vi "Teste de resolução.vi"() -> ()   [LabVIEW 2020]
uses:
  <vilib>/vision/NI_Vision_Development_Module.lvlib
panel:
  in  "Pasta das imagens":path
  in  "Fonte das imagens":enum16{"Imagens na pasta", "Câmera"}(ring)
  in  "Resolução":T1(ring)
  in  "Código para rastrear":enum16{"QR Code", "Data Matrix"}(ring)
  in  "Altura":u16(slide)=3036 scale=10.0..3036.0
  in  "Largura":u16(slide)=4024 scale=10.0..4024.0
  in  "Stop (F)":bool
  out "Image Out":T2(plugin-control)
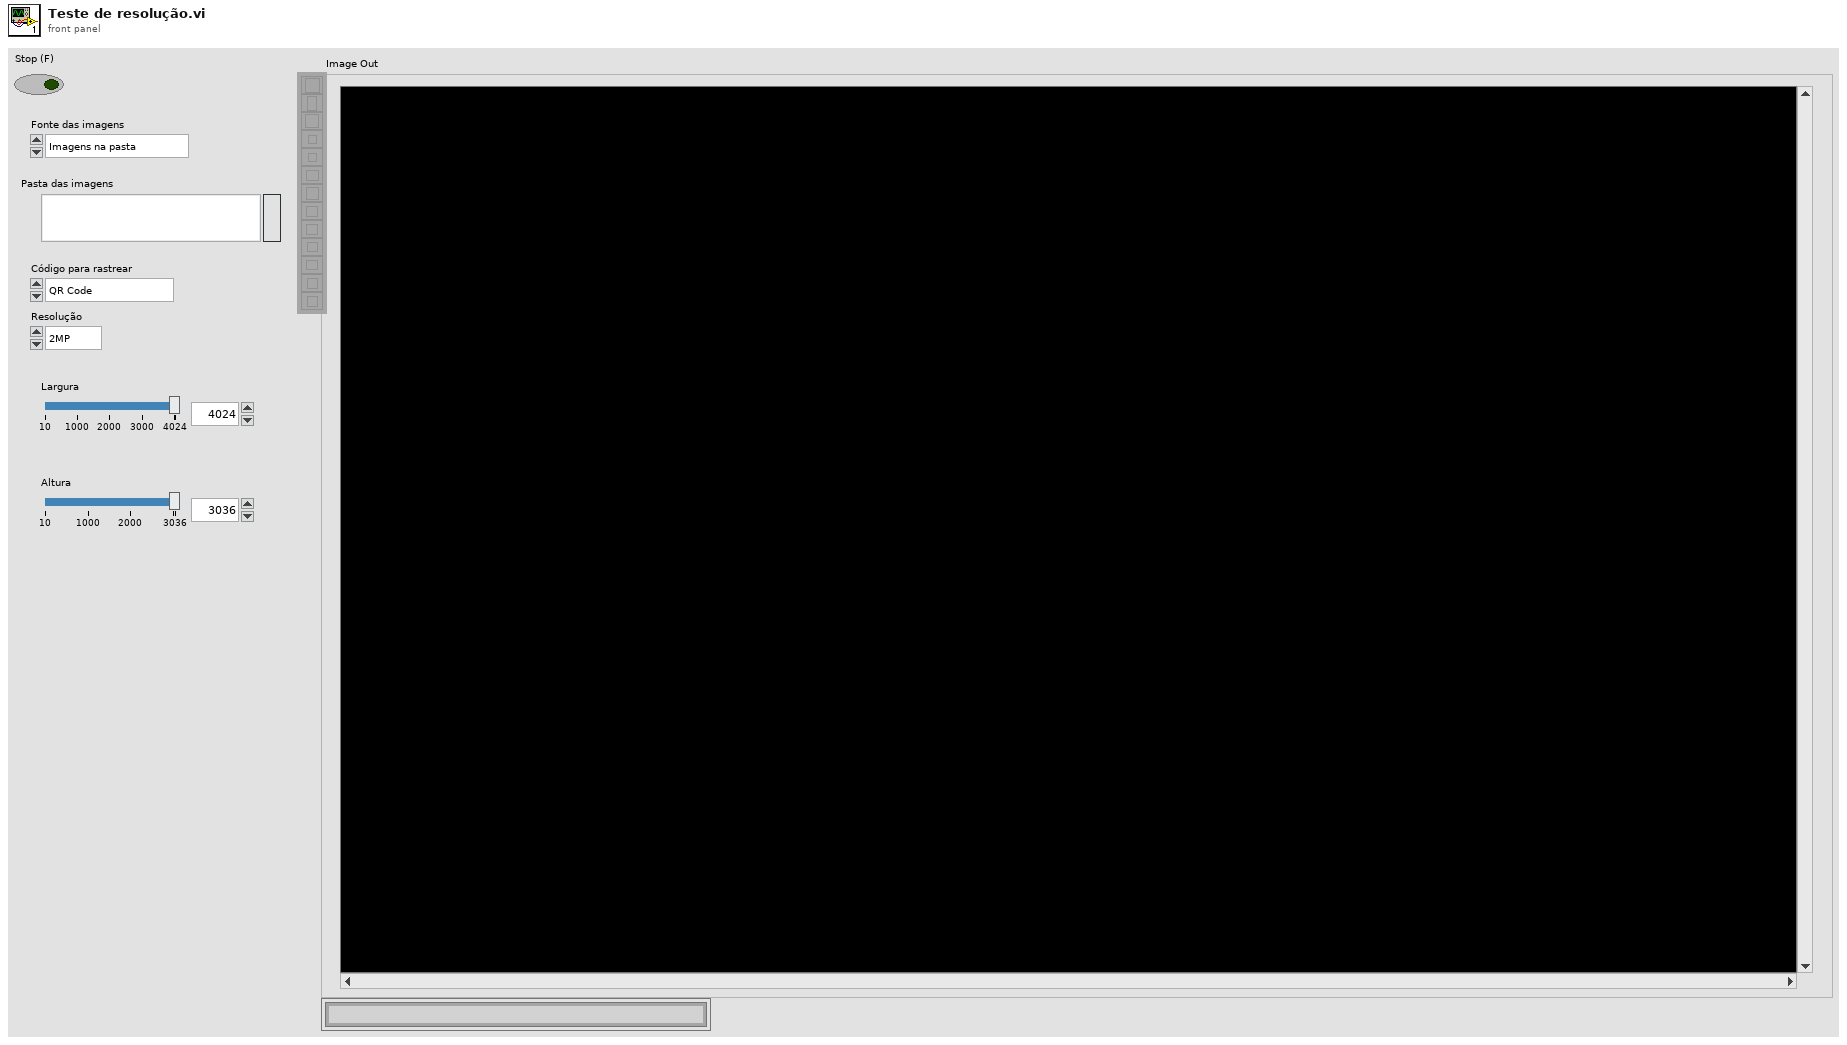
[diagram p1: front panel]
types:
  T1 = enum16{"2MP", "3MP", "5MP", "7MP", "8MP", "10MP", "12MP"}
  T2 = typedef "IMAQ Image.ctl" = refnum<image>
  T3 = cluster{"Global Rectangle":i32[], "Contours":cluster{"Contour Type":u32, "ROI Type":u32, "Points":i32[]}[]}
  T4 = typedef "QR Code Report.ctl" = cluster{"Found?":bool, "Data":string, "Bounding Box":cluster{"x":sgl, "y":sgl}[], "Errors Corrected":u32, "Dimensions (Rows/Cols)":u32, "Version":u32, "QR Model":T5, "Stream Mode":T6, "Barcode Polarity":T7, "Mirrored?":bool, "Append Stream Position":u32, "Size of Append Stream":u32, "First EAN-128 ID":i32, "First Alternate Language ID":i32, "Append Stream ID":u32, "Minimum Edge Strength":u32, "Demodulation Mode":T8, "Cell Sample Size":T9, "Cell Filter Mode":T10}
  T5 = typedef "QR Code Model Type.ctl" = i32
  T6 = typedef "QR Code Stream Mode Type.ctl" = i32
  T7 = typedef "Data Matrix Polarity.ctl" = i32
  T8 = typedef "Demodulation Mode.ctl" = i32
  T9 = typedef "Cell Sample Size.ctl" = i32
  T10 = typedef "Cell Filter Mode.ctl" = i32
  T11 = typedef "Data Matrix Report.ctl" = cluster{"Found?":bool, "Binary?":bool, "Data":string, "Bounding Box":cluster{"x":sgl, "y":sgl}[], "Errors Corrected":u32, "Erasures Corrected":u32, "Aspect Ratio":sgl, "Rows":u32, "Columns":u32, "ECC":T12, "Barcode Polarity":T7, "Cell Fill Percentage":T13, "Border Integrity":sgl, "Mirrored?":bool, "Minimum Edge Strength":u32, "Demodulation Mode":T8, "Cell Sample Size":T9, "Cell Filter Mode":T10, "Iterations":u32}
  T12 = typedef "ECC Type.ctl" = i32
  T13 = typedef "Cell Fill Percentage.ctl" = i32
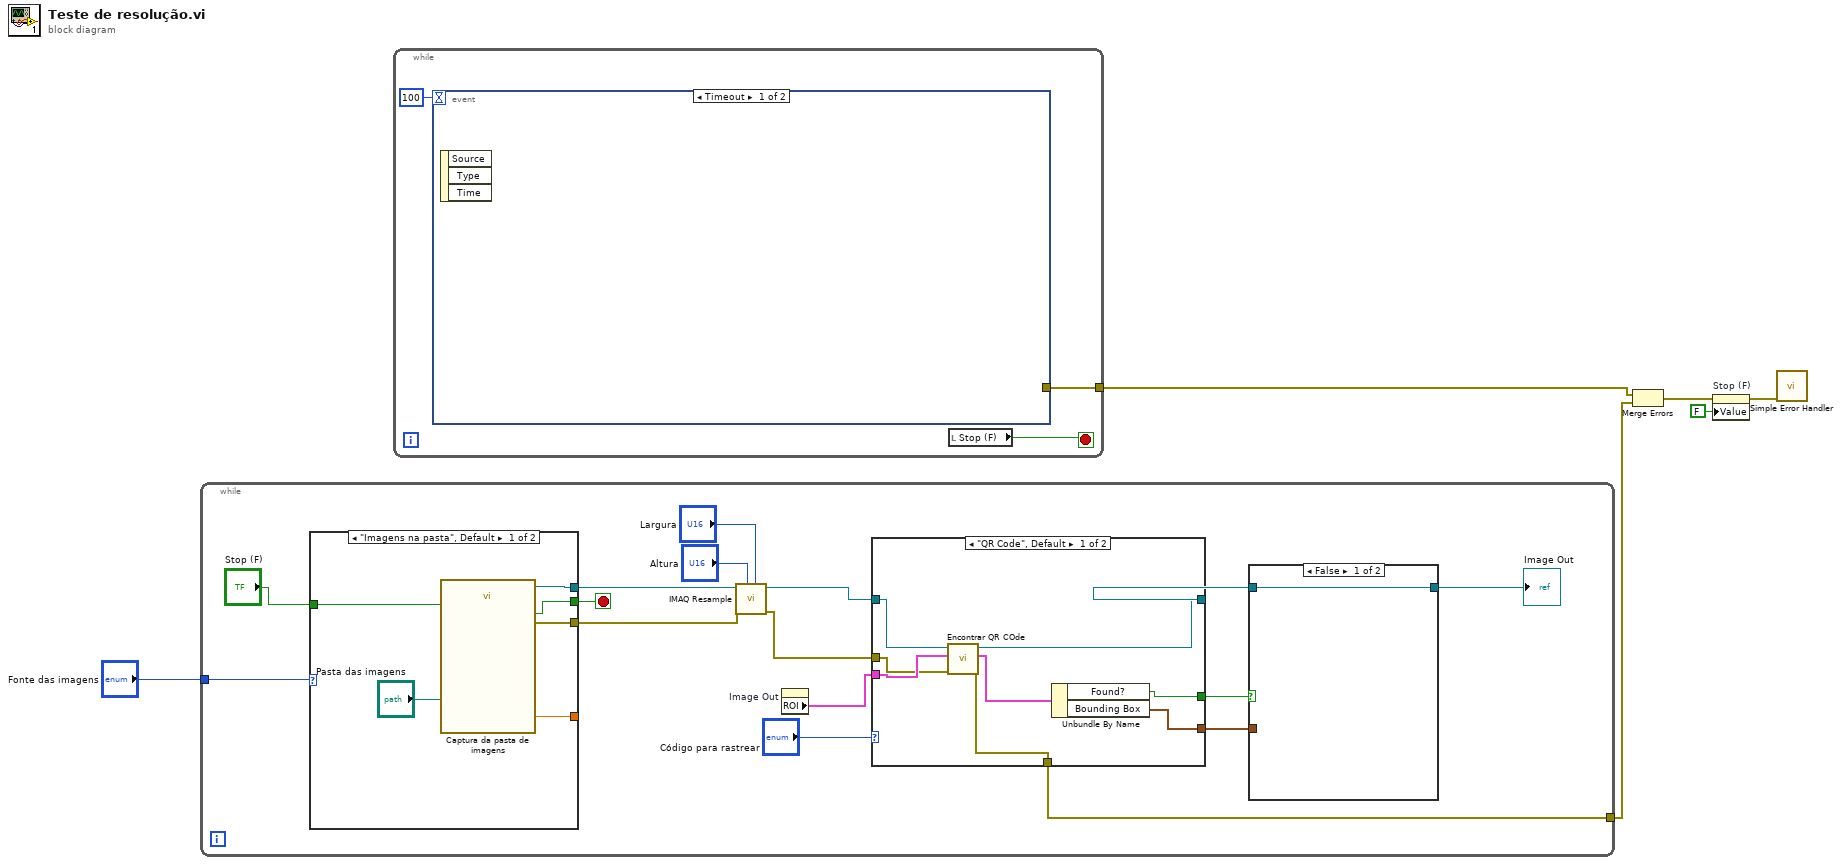
[diagram p0: block diagram]
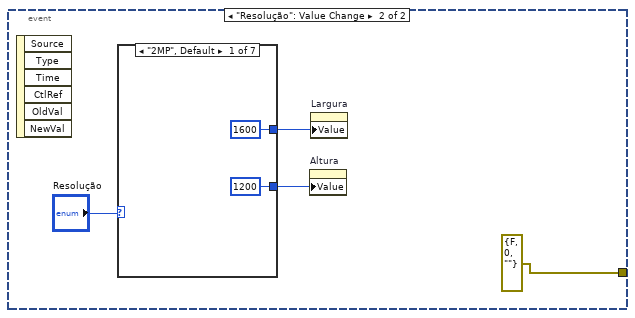
[diagram p2: hidden frame]
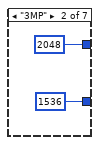
[diagram p3: hidden frame]
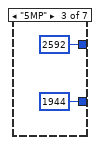
[diagram p4: hidden frame]
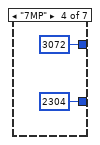
[diagram p5: hidden frame]
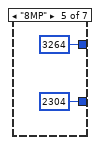
[diagram p6: hidden frame]
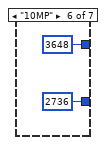
[diagram p7: hidden frame]
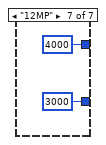
[diagram p8: hidden frame]
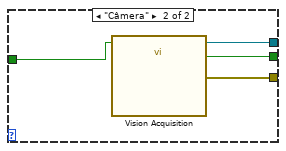
[diagram p9: hidden frame]
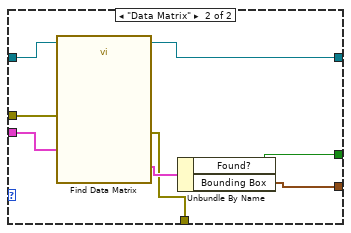
[diagram p10: hidden frame]
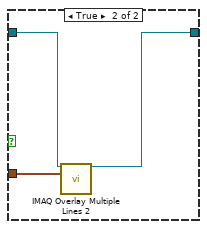
[diagram p11: hidden frame]
diagram:
  n1 = while {
    tunnel: [w10] -> w4
    tunnel: "Fonte das imagens" -> [w9]
    stop <- w8 stop-if-true
    n2 = case shown="\"Imagens na pasta\", Default" w9 {
      tunnel: [w24 w32] -> w8
      tunnel: [w27 w31] -> w19
      tunnel: [w28 w30] -> w17
      tunnel: [w25 _] -> _
      tunnel: "Stop (F)" -> [w23 w29]
      frame "Imagens na pasta", Default {
        n3 = call "Captura da pasta de imagens"("Image Path"="Pasta das imagens", "Stop (F)"=w23) -> ("Image Out"=w27:T2, "Frame Rate"=w25:dbl, "Stopped"=w24:bool, "error out"=w28:errorcluster)  [unwired: 21 in, 1 out]
      }
      frame "Câmera" {
        n4 = call "Vision Acquisition"("Stop (F)"=w29) -> ("Image Out"=w31:T2, "Stopped"=w32:bool, "error out"=w30:errorcluster)  [unwired: 24 in]
      }
    }
    n5 = call "IMAQ Resample"("X Resolution"="Largura", "Y Resolution"="Altura", "error in (no error)"=w17, "Image Src"=w19) -> ("error out"=w16:errorcluster, "Image Dst Out"=w18:T2)  [unwired: 6 in]
    n6 = property on="Image Out" class="ImageControl"() -> ("ROI"=w22:T3)  [unwired: 2 in, 2 out]
    n7 = case shown="\"QR Code\", Default" "Código para rastrear" {
      tunnel: w22 -> [w40 w48]
      tunnel: [w39 w47] -> w21
      tunnel: w18 -> [w38 w46]
      tunnel: w16 -> [w37 w45]
      tunnel: [w35 w43] -> w12
      tunnel: [w34 w42] -> w11
      tunnel: [w33 w41] -> w10
      frame "QR Code", Default {
        n8 = call "Encontrar QR COde.vi"("error in (no error)"=w37, "ROI"=w40, "Refnum in"=w38) -> ("error out"=w33:errorcluster, "QR Barcode Report (QR Code)"=w36:T4, "Refnum out"=w39:T2)  [unwired: 6 in]
        n9 = Unbundle By Name(w36) -> ("Found?"=w35:bool, "Bounding Box"=w34:cluster{"x":sgl, "y":sgl}[])
      }
      frame "Data Matrix" {
        n10 = call "Find Data Matrix"("Image In"=w46, "ROI Descriptor (Data Matrix)"=w48, "error in"=w45) -> ("Image Out"=w47:T2, "Barcode Report (Data Matrix)"=w44:T11, "error out"=w41:errorcluster)  [unwired: 22 in]
        n11 = Unbundle By Name(w44) -> ("Found?"=w43:bool, "Bounding Box"=w42:cluster{"x":sgl, "y":sgl}[])
      }
    }
    n12 = case shown="False" w12 {
      tunnel: w11 -> [_ w52]
      tunnel: w21 -> [w49 w51]
      tunnel: [w49 w50] -> w20
      frame False {
      }
      frame True {
        n13 = call "IMAQ Overlay Multiple Lines 2"("Image"=w51, "Line End Points"=w52) -> ("Image Out"=w50:T2)  [unwired: 12 in, 1 out]
      }
    }
    "Image Out" <- w20
  }
  n14 = while {
    tunnel: [w54] -> w3
    stop <- w55 stop-if-true
    n15 = event shown="[0] Timeout" {
      selector: _ -> [_ _]
      dyn-events: _ -> [_ _]
      timeout: 100 -> [_ _]
      tunnel: [_ errorcluster {"status"=FALSE, "code"=0, "source"=""} ("error constant")] -> w54
      event Timeout {
        n16 = event-data() -> ()  [unwired: 1 in, 3 out]
      }
      event "Resolução": Value Change {
        n17 = event-data() -> ()  [unwired: 1 in, 6 out]
        n18 = case shown="\"2MP\", Default" "Resolução" {
          tunnel: [u16 1600 ("Largura") u16 2048 ("Largura") u16 2592 ("Largura") u16 3072 ("Largura") u16 3264 ("Largura") u16 3648 ("Largura") u16 4000 ("Largura")] -> w58
          tunnel: [u16 1200 ("Altura") u16 1536 ("Altura") u16 1944 ("Altura") u16 2304 ("Altura") u16 2304 ("Altura") u16 2736 ("Altura") u16 3000 ("Altura")] -> w57
          frame "2MP", Default {
          }
          frame "3MP" {
          }
          frame "5MP" {
          }
          frame "7MP" {
          }
          frame "8MP" {
          }
          frame "10MP" {
          }
          frame "12MP" {
          }
        }
        n19 = property on="Altura" class="Slide (strict)"("Value"=w57) -> ()  [unwired: 2 in, 2 out]
        n20 = property on="Largura" class="Slide (strict)"("Value"=w58) -> ()  [unwired: 2 in, 2 out]
      }
    }
    n21 = local read "Stop (F)"() -> (w55:bool)
  }
  n22 = Merge Errors(w3, w4) -> (w5:errorcluster)
  n23 = property on="Stop (F)" class="Bool (strict)"(error in=w5, "Value"=FALSE) -> (error out=w1:errorcluster)  [unwired: 1 in, 1 out]
  n24 = call <vilib>:"Simple Error Handler.vi"("error in (no error)"=w1) -> ()  [unwired: 4 in, 5 out]
